vi "Write and Read Multiple Holding Registers.vi"(4 "read count":u16, 6 "read operation starting address":u16, 8 "error in (no error)":errorcluster, 9 "values to write":u16[](array[numeric]), 10 "write operation starting address":u16, 11 "Modbus master in":refnum<class "Modbus Master.lvclass">) -> (0 "error out":errorcluster, 1 "values read":u16[](array[numeric]), 3 "Modbus master out":refnum<class "Modbus Master.lvclass">)   [LabVIEW 2018, in "Modbus Master.lvclass"]
doc: "Writes and reads values to and from contiguous holding registers. This VI performs the write operation before the read operation. The maximum number of holding registers this VI can write is 121. The maximum number of holding registers this VI can read is 125."
uses:
  Modbus Master.lvclass
  C:/Program Files (x86)/National Instruments/LabVIEW 2018/vi.lib/Modbus/subvis/Modbus API/Modbus API.lvclass
  Modbus API.lvclass/Modbus API.ctl
  Modbus Master.lvclass/Modbus Master.ctl
  Network Master.lvclass
  C:/Program Files (x86)/National Instruments/LabVIEW 2018/vi.lib/Modbus/subvis/Protocol/Interfaces/Network Protocol/Network Protocol.lvclass
  Transmission Data Unit.lvclass
  Master Function Definition.lvlib
  Modbus API.lvclass
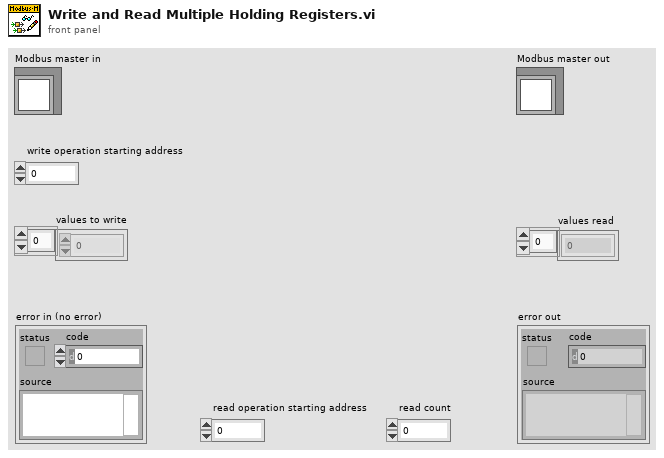
[diagram p1: front panel]
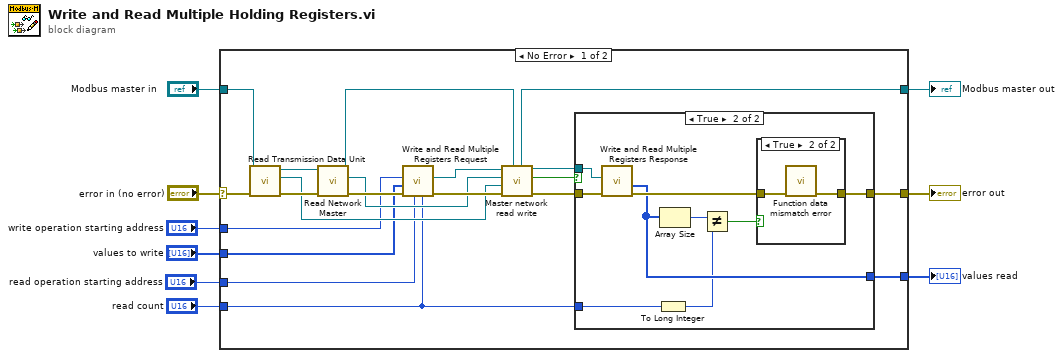
[diagram p0: block diagram]
diagram:
  n1 = case shown="No Error" "error in (no error)" {
    selector: "error in (no error)" -> [w10 w43]
    tunnel: "Modbus master in" -> [w11 w44]
    tunnel: [w24 w44] -> w8
    tunnel: [w28 w43] -> w7
    tunnel: "read count" -> [w17 _]
    tunnel: [w16 _] -> w4
    tunnel: "read operation starting address" -> [w15 _]
    tunnel: "values to write" -> [w14 _]
    tunnel: "write operation starting address" -> [w13 _]
    frame No Error {
      n2 = call "Read Transmission Data Unit.vi"("error in (no error)"=w10, "Modbus instance in"=w11) -> ("error out"=w22:errorcluster, "transmission data unit"=w19:refnum<class "Transmission Data Unit.lvclass">, "Modbus instance out"=w23:refnum<class "Modbus Master.lvclass">)  [unwired: 7 in]
      n3 = call "Read Network Master.vi"("error in (no error)"=w22, "Modbus master in"=w23) -> ("error out"=w21:errorcluster, "network master"=w18:refnum<class "Network Master.lvclass">, "Modbus master out"=w20:refnum<class "Modbus Master.lvclass">)  [unwired: 7 in]
      n4 = call "Write and Read Multiple Registers Request.vi"("quantity to read"=w17, "read starting address"=w15, "error in (no error)"=w21, "write"=w14, "write starting address"=w13) -> ("error out"=w29:errorcluster, "Modbus data unit out"=w26:refnum<class "Modbus Data Unit (PDU).lvclass">)  [unwired: 5 in]
      n5 = call "Master network read write.vi"("Modbus master in"=w20, "error in (no error)"=w29, "transmission data unit in"=w19, "network master in"=w18, "Modbus data unit in"=w26) -> ("error out"=w27:errorcluster, "PDU valid?"=w12:bool, "Modbus data unit out"=w25:refnum<class "Modbus Data Unit (PDU).lvclass">, "Modbus master out"=w24:refnum<class "Modbus Master.lvclass">)  [unwired: 3 in]
      n6 = case shown="True" w12 {
        tunnel: [w30 w39] -> w28
        tunnel: w27 -> [w30 w38]
        tunnel: w25 -> [_ w37]
        tunnel: w17 -> [_ w33]
        tunnel: [_ w32] -> w16
        frame False {
        }
        frame True {
          n7 = call "Write and Read Multiple Registers Response.vi"("error in (no error)"=w38, "Modbus data unit in"=w37) -> ("error out"=w36:errorcluster, "registers"=w32:u16[])  [unwired: 7 in, 1 out]
          n8 = To Long Integer(number=w33) -> (32bit integer=w31:i32)
          n9 = Array Size(array=w32) -> (size(s)=w34:i32)
          n10 = Not Equal?(x=w34, y=w31) -> (x != y?=w35:bool)
          n11 = case shown="True" w35 {
            tunnel: [w40 w42] -> w39
            tunnel: w36 -> [w40 w41]
            frame False {
            }
            frame True {
              n12 = call "Function data mismatch error.vi"("error in (no error)"=w41) -> ("error out"=w42:errorcluster)  [unwired: 10 in]
            }
          }
        }
      }
    }
    frame Error {
    }
  }
  "error out" <- w7
  "Modbus master out" <- w8
  "values read" <- w4
